vi "연속쓰기(Main).vi"() -> ()   [LabVIEW 2014]
panel:
  out "Error":bool
  in  "데이터":u16[](array[numeric])=[13106, 13104, 13107, 13108, 9521, 12848, 13620, 13879] format="%.0x"
  out "데이터 출력":string
  in  "직접변수":string="%DB0000"
  out "에러 출력":errorcluster
  in  "주소":string="192.168.0.10"
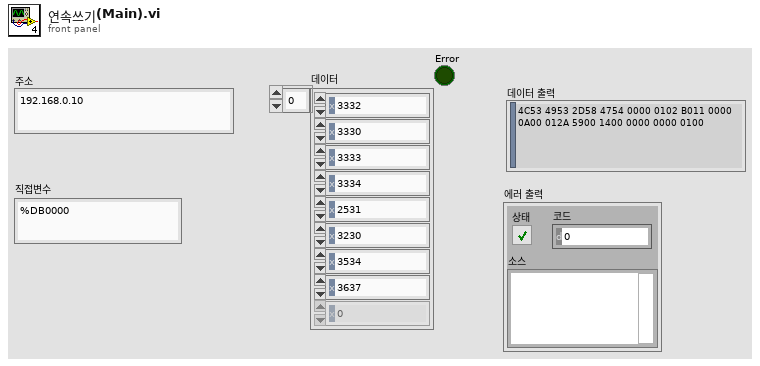
[diagram p1: front panel]
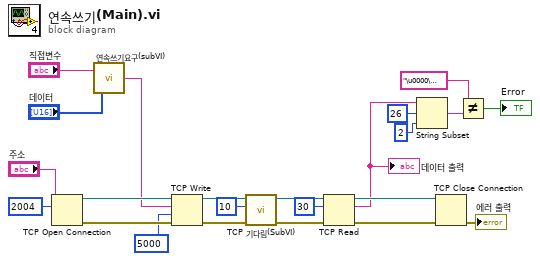
[diagram p0: block diagram]
diagram:
  n1 = TCP Open Connection(address="주소", remote port or service name=u16 2004 ("원격 포트 또는 서비스 이름")) -> (connection ID=w21:refnum<k5>, error out=w20:errorcluster)  [unwired: 3 in]
  n2 = call "연속쓰기요구(subVI).vi"("데이터"="데이터", "직접변수"="직접변수") -> ("연속쓰기"=w14:string)
  n3 = TCP Write(connection ID=w21, data in=w14, error in (no error)=w20, 9:5000 ("타임아웃 ms (25000)")) -> (connection ID out=w13:refnum<k5>, error out=w11:errorcluster)  [unwired: 1 out]
  n4 = call "TCP 기다림(SubVI).vi"("error in"=w11, "기다림(ms)"=u32 10, "TCP 네트워크 연결 입력"=w13) -> ("error out"=w10:errorcluster, "TCP 네트워크 연결 출력"=w12:refnum<k5>)  [unwired: 7 in]
  n5 = TCP Read(connection ID=w12, bytes to read=30 ("읽을 바이트"), error in (no error)=w10) -> (connection ID out=w19:refnum<k5>, data out=w6:string, error out=w18:errorcluster)  [unwired: 2 in]
  "데이터 출력" <- w6
  n6 = String Subset(string=w6, offset (0)=26 ("오프셋(0)"), length (rest)=2 ("길이(나머지)")) -> (substring=w3:string)
  n7 = TCP Close Connection(connection ID=w19, error in (no error)=w18) -> (error out=→"에러 출력":errorcluster)  [unwired: 1 in, 1 out]
  n8 = Not Equal?(x="\u0000\u0000", y=w3) -> (x != y?=→"Error":bool)
